vi "PushSlideTiles.vi"(8 "error in (no error)":errorcluster, 11 "Game in":refnum<class "Game.lvclass">) -> (0 "error out":errorcluster, 3 "Game out":refnum<class "Game.lvclass">)   [LabVIEW 2019, in "RT_Game.lvlib" / "Game.lvclass"]
uses:
  Game.lvclass
  Game.lvclass/Game.ctl
  Coordinate.ctl
  <vilib>/Utility/error.llb/Error Cluster From Error Code.vi
  <vilib>/rvi/errors/niLvFpgaAdjustHostInterfaceError.vi
  <vilib>/rvi/interface/nirviMethod/nirviMethod.xnode
  FPGA_Interface.ctl
  FPGA Bitfiles/myriogameconsole_FPGATarget_Main_ntsPRcBZGxk.lvbitx
  <vilib>/FPGAPlugInAG/myRIO-1900/niLvFpga_WriteFifo_myRIO-1900.vi
  <vilib>/rvi/errors/niLvFpgaMergeErrorWithErrorCode.vi
panel:
  out "Array 2":u16[](array[numeric])
  out "Array":u16[](array[numeric])
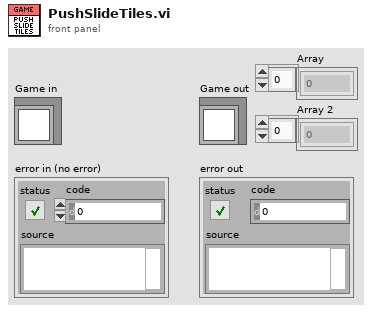
[diagram p1: front panel]
types:
  T1 = typedef "RT_Game.lvlib/Game.lvclass/Coordinate.ctl" = cluster{"x":dbl, "y":dbl}
  T2 = typedef "FPGA_Interface.ctl" = refnum<k20>
  T3 = typedef "RT_Game.lvlib/Engine.lvclass/SlideJob.ctl" = cluster{"Pixel":u32[], "Side":T4}
  T4 = typedef "RT_Game.lvlib/Game.lvclass/ScreenSide.ctl" = enum16{"up", "down", "left", "right", "none"}
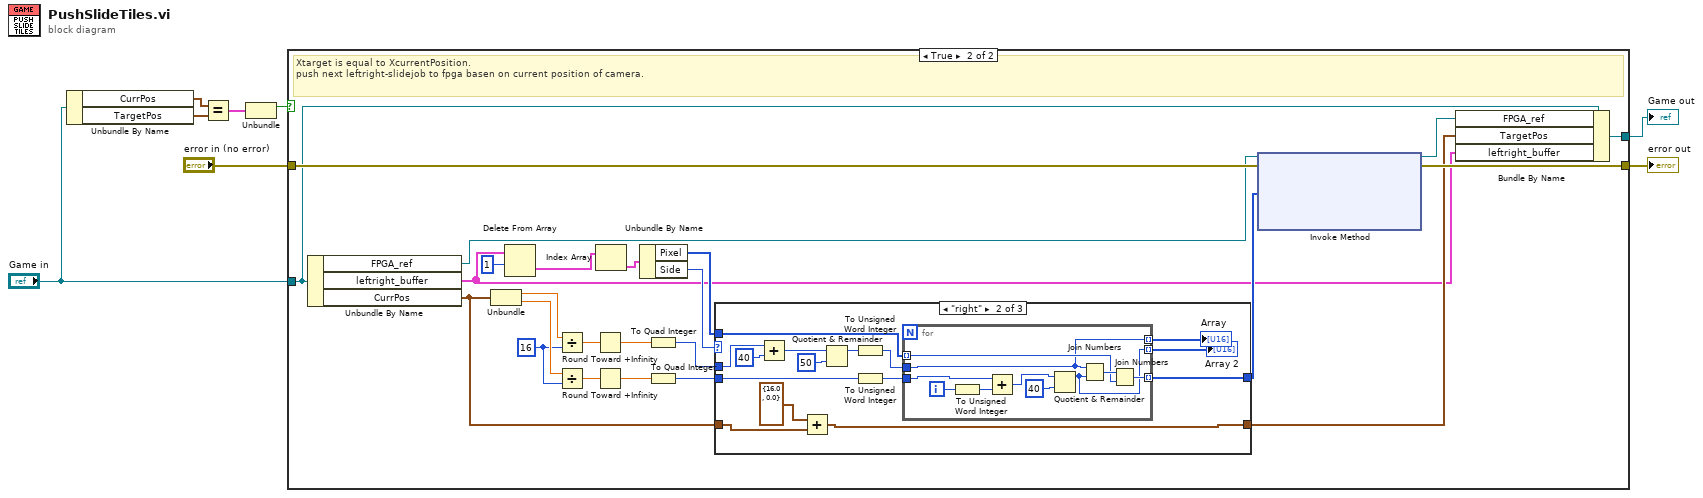
[diagram p0: block diagram]
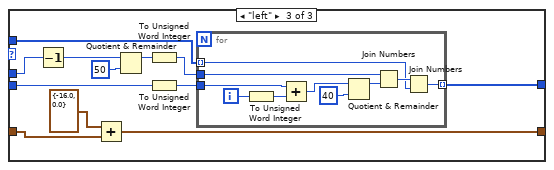
[diagram p4: hidden frame]
diagram:
  n1 = Unbundle By Name("Game in") -> ("CurrPos"=w6:T1, "TargetPos"=w5:T1)
  n2 = Equal?(x=w6, y=w5) -> (x = y?=w4:cluster{"x":bool, "y":bool})
  n3 = Unbundle(w4) -> ("x"=w2:bool)  [unwired: 1 out]
  n4 = case shown="True" w2 {
    tunnel: [w9 w34] -> w8
    tunnel: "error in (no error)" -> [w9 w32]
    tunnel: "Game in" -> [w10 w30]
    tunnel: [w10 w29] -> w7
    frame False {
    }
    frame True {
      w15 = u16 16 ("y")
      # "Xtarget is equal to XcurrentPosition.\npush next leftright-slidejob to fpga basen on current position of camera."
      n5 = Unbundle By Name(w30) -> ("FPGA_ref"=w31:T2, "leftright_buffer"=w11:T3[], "CurrPos"=w12:T1)
      n6 = Unbundle(w12) -> ("x"=w16:dbl, "y"=w21:dbl)
      n7 = Delete From Array(array=w11, length=1) -> (deleted portion=w27:T3[])  [unwired: 1 in, 1 out]
      n8 = Divide(x=w16, y=w15) -> (x/y=w20:dbl)
      n9 = Divide(x=w21, y=w15) -> (x/y=w19:dbl)
      n10 = Round Toward +Infinity(x=w20) -> (ceil(x): smallest int >= x=w18:dbl)
      n11 = Round Toward +Infinity(x=w19) -> (ceil(x): smallest int >= x=w17:dbl)
      n12 = Index Array(array=w27) -> (element=w26:T3)  [unwired: 1 in]
      n13 = Unbundle By Name(w26) -> ("Pixel"=w24:u32[], "Side"=w25:T4)
      n14 = To Quad Integer(1:w18) -> (0:w13:i64)
      n15 = To Quad Integer(1:w17) -> (0:w14:i64)
      n16 = case shown="\"right\"" w25 {
        tunnel: w13 -> [_ w43 w66]
        tunnel: w14 -> [_ w42 w65]
        tunnel: w24 -> [_ w41 w64]
        tunnel: w12 -> [w35 w40 w63]
        tunnel: [w35 w39 w62] -> w23
        tunnel: [_ w38 w61] -> w22
        frame Default {
        }
        frame "right" {
          n17 = Add(x=w43, y=u16 40) -> (x+y=w49:i64)
          n18 = Add(x=T1 {"x"=16.0, "y"=0.0}, y=w40) -> (x+y=w39:T1)
          n19 = Quotient & Remainder(x=w49, y=u16 50) -> (x-y*floor(x/y)=w47:i64)  [unwired: 1 out]
          n20 = To Unsigned Word Integer(number=w47) -> (unsigned 16bit integer=w46:u16)
          n21 = To Unsigned Word Integer(number=w42) -> (unsigned 16bit integer=w45:u16)
          n22 = for {
            tunnel: w45 -> [w58]
            tunnel: w46 -> [w52]
            tunnel: [w54] -> w38 mode=indexing
            tunnel: w41 -> [w53] mode=indexing
            tunnel: [w52] -> w37 mode=indexing
            tunnel: [w51] -> w36 mode=indexing
            i -> [w59]
            n23 = To Unsigned Word Integer(number=w59) -> (unsigned 16bit integer=w55:u16)
            n24 = Add(x=w58, y=w55) -> (x+y=w56:u16)
            n25 = Quotient & Remainder(x=w56, y=u16 40) -> (x-y*floor(x/y)=w51:u16)  [unwired: 1 out]
            n26 = Join Numbers(hi=w52, lo=w51) -> ((hi.lo)=w60:u32)
            n27 = Join Numbers(hi=w60, lo=w53) -> ((hi.lo)=w54:u64)
          }
          "Array" <- w37
          "Array 2" <- w36
        }
        frame "left" {
          n28 = Decrement(x=w66) -> (x-1=w69:i64)
          n29 = Add(x=T1 {"x"=-16.0, "y"=0.0}, y=w63) -> (x+y=w62:T1)
          n30 = Quotient & Remainder(x=w69, y=u16 50) -> (x-y*floor(x/y)=w71:i64)  [unwired: 1 out]
          n31 = To Unsigned Word Integer(number=w71) -> (unsigned 16bit integer=w70:u16)
          n32 = To Unsigned Word Integer(number=w65) -> (unsigned 16bit integer=w68:u16)
          n33 = for {
            tunnel: w68 -> [w80]
            tunnel: w70 -> [w79]
            tunnel: [w74] -> w61 mode=indexing
            tunnel: w64 -> [w73] mode=indexing
            i -> [w81]
            n34 = To Unsigned Word Integer(number=w81) -> (unsigned 16bit integer=w75:u16)
            n35 = Add(x=w80, y=w75) -> (x+y=w77:u16)
            n36 = Quotient & Remainder(x=w77, y=u16 40) -> (x-y*floor(x/y)=w76:u16)  [unwired: 1 out]
            n37 = Join Numbers(hi=w79, lo=w76) -> ((hi.lo)=w82:u32)
            n38 = Join Numbers(hi=w82, lo=w73) -> ((hi.lo)=w74:u64)
          }
        }
      }
      n39 = xnode "Invoke Method"("FPGA VI Reference In"=w31, "error in"=w32, "Data"=w22) -> ("FPGA VI Reference Out"=w33:T2, "error out"=w34:errorcluster)  [unwired: 1 in, 1 out]
      n40 = Bundle By Name(cluster=w30, "FPGA_ref"=w33, "TargetPos"=w23, "leftright_buffer"=w11) -> (w29:refnum<class "Game.lvclass">)
    }
  }
  "Game out" <- w7
  "error out" <- w8
